vi "FindClosestEdge_V1.vi"(9 "Radius":dbl, 10 "Position":cluster{"x":dbl, "y":dbl}, 11 "Input picture":dbl[][](array[numeric])) -> (3 "Position out":cluster{"x":dbl, "y":dbl})   [LabVIEW 2014]
panel:
  out "found relative position":cluster{i32, i32}
  out "Intensity Graph":dbl[][](graph)
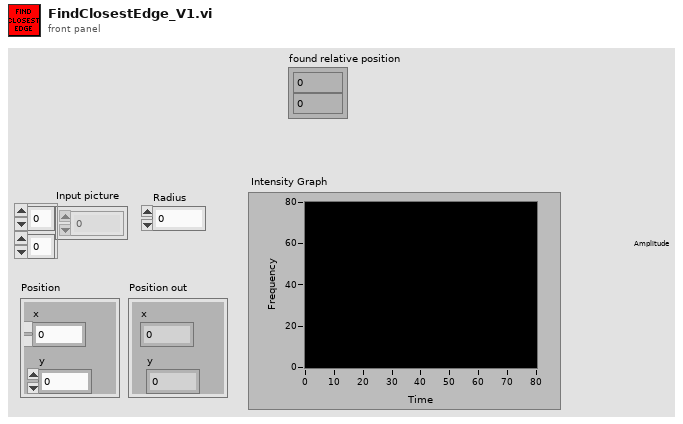
[diagram p1: front panel]
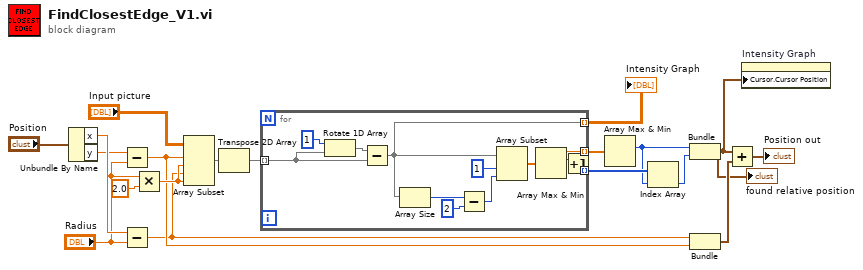
[diagram p0: block diagram]
diagram:
  n1 = Unbundle By Name("Position") -> ("x"=w12:dbl, "y"=w11:dbl)
  n2 = Subtract(x=w11, y="Radius") -> (x-y=w5:dbl)
  n3 = Subtract(x=w12, y="Radius") -> (x-y=w4:dbl)
  n4 = Multiply(x="Radius", y=2.0) -> (x*y=w18:dbl)
  n5 = Array Subset(array="Input picture", index (row)=w5, length (row)=w18, index (col)=w4, length (col)=w18) -> (w6:dbl[][])
  n6 = Transpose 2D Array(2D array=w6) -> (transposed array=w3:dbl[][])
  n7 = for {
    tunnel: w3 -> [w29] mode=indexing
    tunnel: [w23] -> w16 mode=indexing
    tunnel: [w20] -> w15 mode=indexing
    tunnel: [w21] -> w2 mode=indexing
    n8 = Rotate 1D Array(1:w29, 2:1 ("n")) -> (0:w30:dbl[])
    n9 = Subtract(x=w30, y=w29) -> (x-y=w21:dbl[])
    n10 = Array Size(array=w21) -> (size(s)=w28:i32)
    n11 = Subtract(x=w28, y=2) -> (x-y=w26:i32)
    n12 = Array Subset(array=w21, index=1, length=w26) -> (w24:dbl[])
    n13 = Array Max & Min(array=w24) -> (max value=w23:dbl, max index (indices)=w22:i32)  [unwired: 2 out]
    n14 = Increment(x=w22) -> (x+1=w20:i32)
  }
  "Intensity Graph" <- w2
  n15 = Array Max & Min(array=w16) -> (max index (indices)=w13:i32)  [unwired: 3 out]
  n16 = Index Array(array=w15, index=w13) -> (element=w14:i32)
  n17 = Bundle(w13, w14) -> (w1:cluster{i32, i32})  [unwired: 1 in]
  "found relative position" <- w1
  n18 = Bundle(w4, w5) -> (w8:cluster{dbl, dbl})  [unwired: 1 in]
  n19 = Add(x=w1, y=w8) -> (x+y=→"Position out":cluster{dbl, dbl})
  n20 = property on="Intensity Graph" class="IntGraph (strict)"("Cursor.Cursor Position"=w1) -> ()  [unwired: 2 in, 2 out]
